vi "Dropdown - Mouse Up.vi"(0 "Table Ref":refnum<vi>, 5 "Unit Abbreviations":string[](array[string]), 7 "WindowPos":cluster{"Left":i16, "Top":i16}, 9 "Cursor Position":i32[](array[numeric]), 11 "Error In":errorcluster) -> (4 "Dropdown Bundle":T2, 15 "Error Out":errorcluster)   [LabVIEW 2013]
uses:
  <vilib>/Utility/miscctls.llb/LVRowAndColumnTypeDef.ctl
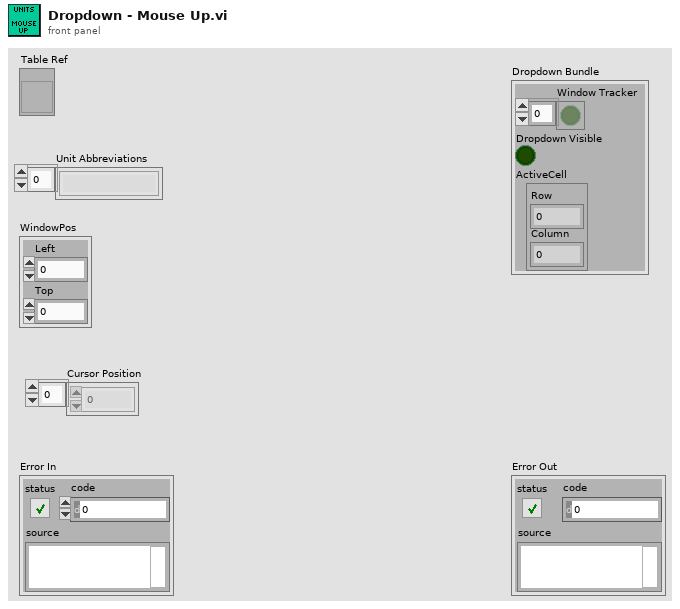
[diagram p1: front panel]
types:
  T1 = typedef "LVRowAndColumnTypeDef.ctl" = cluster{"Row":i32, "Column":i32}
  T2 = cluster{"Window Tracker":bool[], "Dropdown Visible":bool, "ActiveCell":T1}
  T3 = enum16{"Set Abbreviations", "Set Engine Mode", "Set Enum Position", "Get Abbreviation", "Write Abbreviation", "Read Enum Position", "Read Engine Mode", "Read Abbreviations", "Engine Started", "Check Engine", "Init Global", "Set Cursor", "Read Cursor"}
  T4 = enum16{"Idle", "Reveal Dropdown", "Hide FP", "Set Options"}
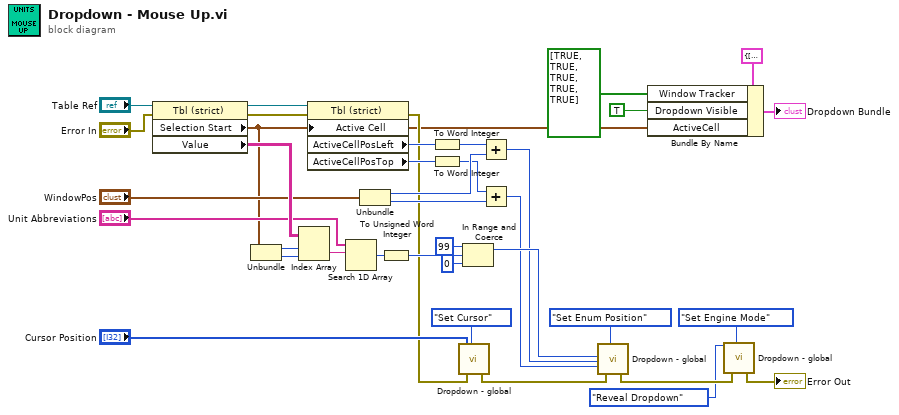
[diagram p0: block diagram]
diagram:
  n1 = property on="Property Node" class="Tbl (strict)"(reference="Table Ref", error in="Error In") -> (reference out=w27:refnum<vi>, error out=w29:errorcluster, "Selection Start"=w1:T1, "Value"=w23:string[][])
  n2 = Unbundle(w1) -> ("Row"=w22:i32, "Column"=w21:i32)
  n3 = Index Array(array=w23, index (row)=w22, index (col)=w21) -> (element=w24:string)
  n4 = property on="Property Node" class="Tbl (strict)"(reference=w27, error in=w29, "Active Cell"=w1) -> (error out=w7:errorcluster, "ActiveCellPosLeft"=w12:i32, "ActiveCellPosTop"=w9:i32)  [unwired: 1 out]
  n5 = Search 1D Array(1D array="Unit Abbreviations", element=w24) -> (index of element=w18:i32)  [unwired: 1 in]
  n6 = Unbundle("WindowPos") -> ("Left"=w16:i16, "Top"=w15:i16)
  n7 = To Unsigned Word Integer(number=w18) -> (unsigned 16bit integer=w17:u16)
  n8 = To Word Integer(number=w12) -> (16bit integer=w11:i16)
  n9 = To Word Integer(number=w9) -> (16bit integer=w10:i16)
  n10 = call "Dropdown - global.vi"("Cursor Pos In"="Cursor Position", "Error In"=w7, "Global Mode"=T3."Set Cursor") -> ("Error Out"=w37:errorcluster)  [unwired: 8 in, 8 out]
  n11 = In Range and Coerce(upper limit=u16 99, x=w17, lower limit=u16 0) -> (coerced(x)=w19:u16)  [unwired: 1 out]
  n12 = Add(x=w11, y=w16) -> (x+y=w13:i16)
  n13 = Add(x=w10, y=w15) -> (x+y=w14:i16)
  n14 = call "Dropdown - global.vi"("Ring Index In"=w19, "Left In"=w13, "Top In"=w14, "Error In"=w37, "Global Mode"=T3."Set Enum Position") -> ("Error Out"=w35:errorcluster)  [unwired: 6 in, 8 out]
  n15 = Bundle By Name(cluster=T2 {"Window Tracker"=[], "Dropdown Visible"=FALSE, "ActiveCell"={"Row"=0, "Column"=0}} ("Dropdown Bundle"), "Window Tracker"=bool[] [TRUE, TRUE, TRUE, TRUE, TRUE], "Dropdown Visible"=TRUE, "ActiveCell"=w1) -> (→"Dropdown Bundle":T2)
  n16 = call "Dropdown - global.vi"("Engine Mode In"=T4."Reveal Dropdown", "Error In"=w35, "Global Mode"=T3."Set Engine Mode") -> ("Error Out"=→"Error Out":errorcluster)  [unwired: 8 in, 8 out]
